vi "Configure AWGN Noise.vi"(0 "VISA resource name":refnum<visa-resource-name>, 1 "Auto Noise Integration Bandwidth (T: Enable)":bool=TRUE, 2 "Enable AWGN (T: Enable)":bool=TRUE, 5 "Flat Noise Bandwidth (1 Hz)":dbl=1.0, 7 "Noise Integration Bandwidth (1 Hz)":dbl=1.0, 9 "Additive Noise Control Mode (0: Sum)":i32(ring) items=["Sum", "Signal", "Noise"], 11 "error in (no error)":errorcluster, 12 "Signal/Noise Ratio (0)":dbl) -> (4 "VISA resource name out":refnum<visa-resource-name>, 15 "error out":errorcluster)   [LabVIEW 2018, in "Agilent PSG MXG Series.lvlib"]
doc: "Configrue AWGN noise settings.\n\n<B>Notes:</B>\n(1) This VI is valid only in N5172B with <B>Option 653</B> or <B>Option 655</B>, N5182B with <B>Option 656</B> or <B>Option 657</B>."
uses:
  Agilent PSG MXG Series.lvlib
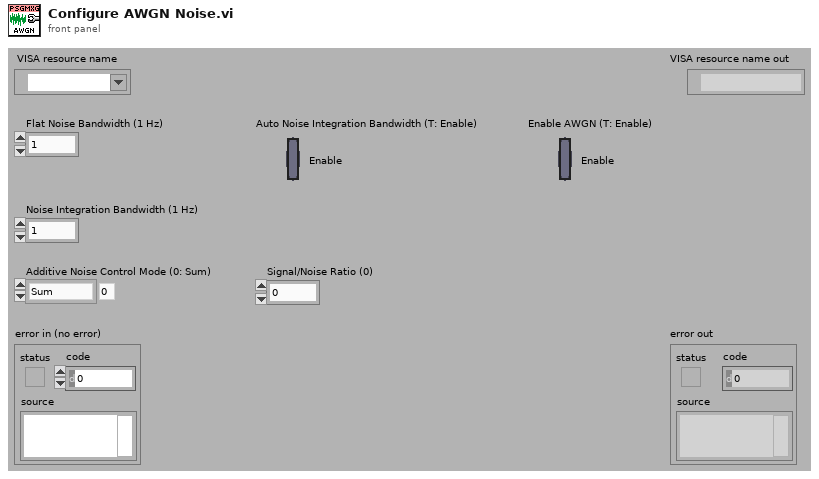
[diagram p1: front panel]
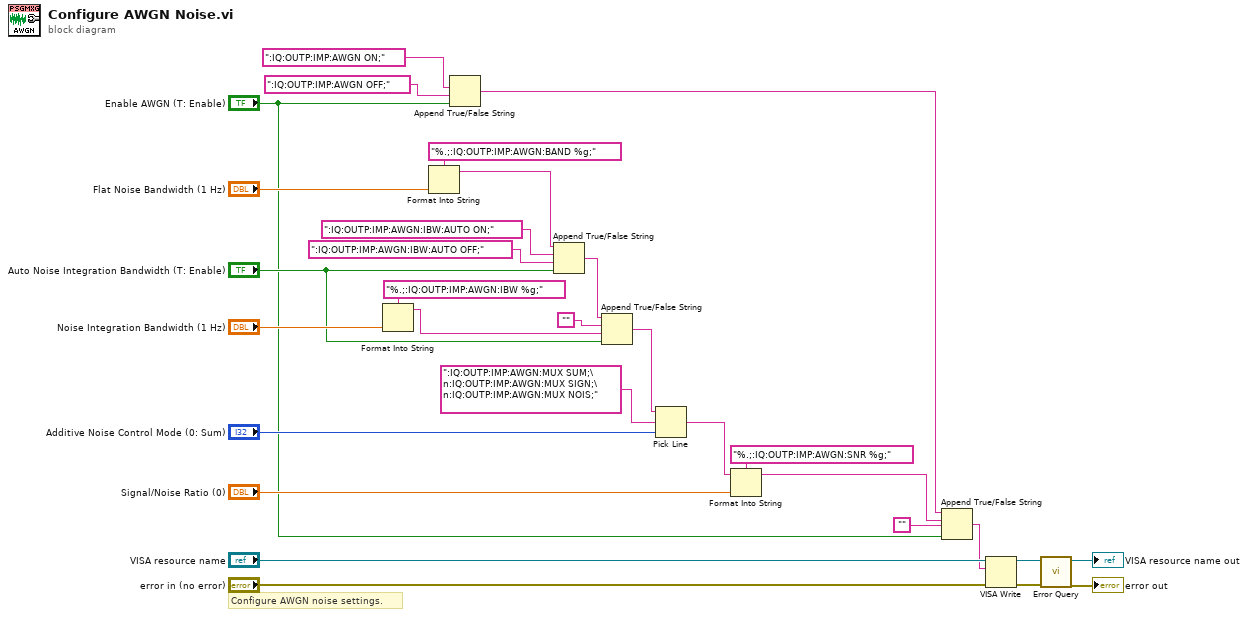
[diagram p0: block diagram]
diagram:
  # "Configure AWGN noise settings."
  n1 = Format Into String(format string="%.;:IQ:OUTP:IMP:AWGN:IBW %g;", "Noise Integration Bandwidth (1 Hz)") -> (resulting string=w8:string)  [unwired: 2 in, 1 out]
  n2 = Format Into String(format string="%.;:IQ:OUTP:IMP:AWGN:BAND %g;", "Flat Noise Bandwidth (1 Hz)") -> (resulting string=w10:string)  [unwired: 2 in, 1 out]
  n3 = Append True/False String(1:"Enable AWGN (T: Enable)", 2:":IQ:OUTP:IMP:AWGN OFF;", 3:":IQ:OUTP:IMP:AWGN ON;") -> (0:w3:string)  [unwired: 1 out]
  n4 = Append True/False String(1:"Auto Noise Integration Bandwidth (T: Enable)", 2:":IQ:OUTP:IMP:AWGN:IBW:AUTO OFF;", 3:":IQ:OUTP:IMP:AWGN:IBW:AUTO ON;", 4:w10) -> (0:w9:string)
  n5 = Append True/False String(1:"Auto Noise Integration Bandwidth (T: Enable)", 2:w8, 3:"", 4:w9) -> (0:w6:string)
  n6 = Pick Line(string ("")=w6, multi-line string=":IQ:OUTP:IMP:AWGN:MUX SUM;\n:IQ:OUTP:IMP:AWGN:MUX SIGN;\n:IQ:OUTP:IMP:AWGN:MUX NOIS;", line index="Additive Noise Control Mode (0: Sum)") -> (output string=w22:string)
  n7 = Format Into String(format string="%.;:IQ:OUTP:IMP:AWGN:SNR %g;", initial string=w22, "Signal/Noise Ratio (0)") -> (resulting string=w2:string)  [unwired: 1 in, 1 out]
  n8 = Append True/False String(1:"Enable AWGN (T: Enable)", 2:"", 3:w2, 4:w3) -> (0:w5:string)
  n9 = VISA Write(VISA resource name="VISA resource name", write buffer=w5, error in (no error)="error in (no error)") -> (VISA resource name out=w15:refnum<visa-resource-name>, error out=w14:errorcluster)  [unwired: 1 out]
  n10 = call "Error Query.vi"("error in (no error)"=w14, "VISA resource name"=w15) -> ("error out"=→"error out":errorcluster, "VISA resource name out"=→"VISA resource name out":refnum<visa-resource-name>)  [unwired: 8 out]
